vi "Empty Table by Reference.vi"(8 "error in (no error)":errorcluster, 11 "Table Control in":refnum<vi>) -> (0 "error out":errorcluster)   [LabVIEW 2021, in "CIF_UI.lvclass"]
uses:
  CIF_UI.lvclass
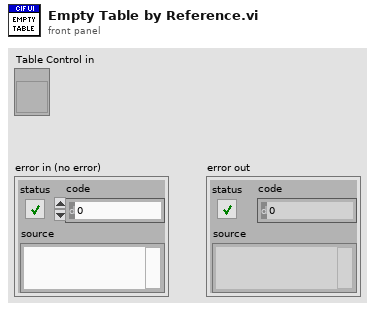
[diagram p1: front panel]
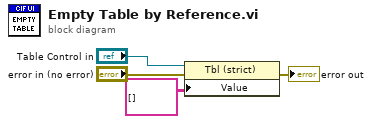
[diagram p0: block diagram]
diagram:
  n1 = property on="Property Node" class="Tbl (strict)"(reference="Table Control in", error in="error in (no error)", "Value"=string[][] []) -> (error out=→"error out":errorcluster)  [unwired: 1 out]
